vi "SNTP Light ActionVIs OnSave.vi"(8 "error in (no error)":errorcluster, 11 "Node Ptr":T1 format="%.0x") -> (0 "error out":errorcluster, 3 "Node Ptr 2":T1=18446744073709551615 format="%.0x")   [LabVIEW 2013, in "SNTP Light Custom Device Configuration.lvlib"]
uses:
  SNTP Light Custom Device Configuration.lvlib
  <vilib>/NI Veristand/Custom Device API/Custom Device API.lvlib
  NationalInstruments.VeriStand.SystemStorage
  NationalInstruments.VeriStand.SystemDefinitionAPI
  <vilib>/NI Veristand/Custom Device API/Custom Device Item Ref.ctl
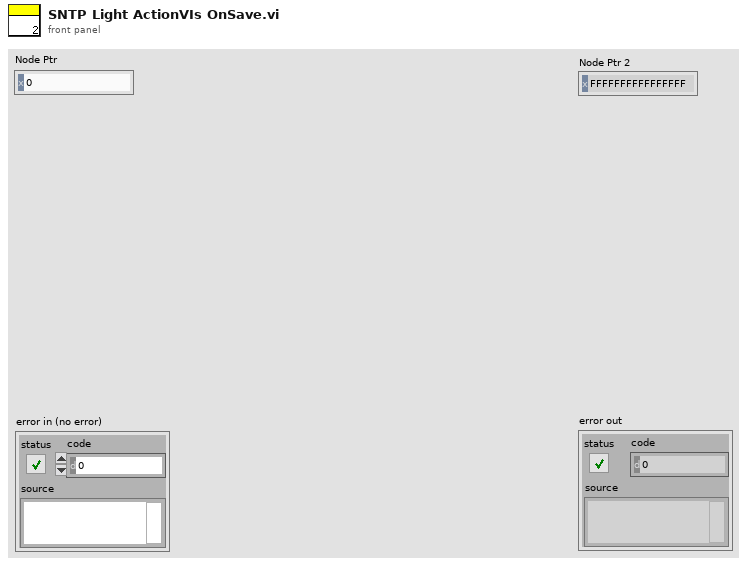
[diagram p1: front panel]
types:
  T1 = typedef "Custom Device API.lvlib/Custom Device Item Ref.ctl" = u64
  T2 = typedef "Custom Device API.lvlib/Custom Device Pointer.ctl" = refnum<k24>
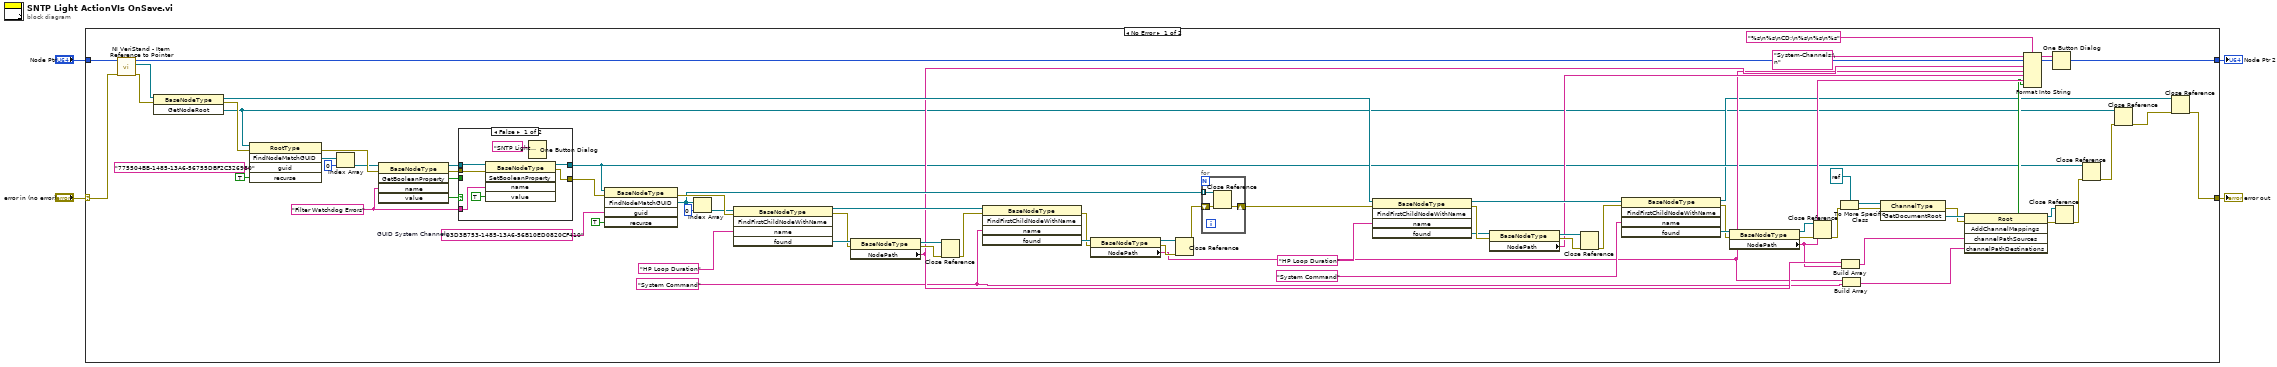
[diagram p0: block diagram]
diagram:
  n1 = case shown="No Error" "error in (no error)" {
    selector: "error in (no error)" -> [w79 w94]
    tunnel: [w74 w94] -> w3
    tunnel: "Node Ptr" -> [w80 w93]
    tunnel: [w76 w93] -> w1
    frame No Error {
      w16 = "System Command" ("name")
      w63 = "03D3B753-1485-13A6-56B10ED0820CF410"  # GUID System Channels
      w64 = "Filter Watchdog Errors" ("name")
      n2 = call <vilib>:"NI VeriStand - Item Reference to Pointer.vi"("error in (no error)"=w79, "Item Ref in"=w80) -> ("error out"=w77:errorcluster, "Node Pointer"=w78:T2, "Item Ref out"=w76:T1)  [unwired: 6 in, 1 out]
      n3 = invoke class="BaseNodeType" method="GetNodeRoot"(reference=w78, error in=w77) -> (reference out=w31:T2, error out=w73:errorcluster, "GetNodeRoot"=w5:refnum<k24>)  [unwired: 1 in]
      n4 = invoke class="RootType" method="FindNodeMatchGUID"(reference=w5, error in=w73, "guid"="775504BB-1485-13A6-56755DBF2C326980", "recurse"=TRUE) -> (error out=w70:errorcluster, "FindNodeMatchGUID"=w69:refnum<k24>[])  [unwired: 1 in, 3 out]
      n5 = Index Array(array=w69, index=0) -> (element=w28:refnum<k24>)
      n6 = invoke class="BaseNodeType" method="GetBooleanProperty"(reference=w28, error in=w70, "name"=w64) -> (reference out=w66:refnum<k24>, error out=w65:errorcluster, "GetBooleanProperty"=w75:bool, "value"=w67:bool)  [unwired: 2 in, 1 out]
      n7 = case shown="False" w67 {
        tunnel: w75 -> [_ _]
        tunnel: w66 -> [w90 w92]
        tunnel: [w89 w92] -> w13
        tunnel: w65 -> [w88 w91]
        tunnel: [w87 w91] -> w62
        tunnel: w64 -> [w86 _]
        frame False {
          n8 = invoke class="BaseNodeType" method="SetBooleanProperty"(reference=w90, error in=w88, "name"=w86, "value"=TRUE) -> (reference out=w89:refnum<k24>, error out=w87:errorcluster)  [unwired: 1 in, 3 out]
          n9 = One Button Dialog(message="SNTP Light Custom Device: \"Filter Watchdog Errors\" Controller Property forced to TRUE.") -> ()  [unwired: 1 in, 1 out]
        }
        frame True {
        }
      }
      n10 = invoke class="BaseNodeType" method="FindNodeMatchGUID"(reference=w13, error in=w62, "guid"=w63, "recurse"=TRUE) -> (error out=w59:errorcluster, "FindNodeMatchGUID"=w44:refnum<k24>[])  [unwired: 1 in, 3 out]
      n11 = Index Array(array=w44, index=0) -> (element=w30:refnum<k24>)
      n12 = invoke class="BaseNodeType" method="FindFirstChildNodeWithName"(reference=w30, error in=w59, "name"="HP Loop Duration") -> (reference out=w57:refnum<k24>, error out=w55:errorcluster, "found"=w56:refnum<k24>)  [unwired: 2 in, 2 out]
      n13 = property class="BaseNodeType"(reference=w56, error in=w55) -> (reference out=w54:refnum<k24>, error out=w53:errorcluster, "NodePath"=w18:string)
      n14 = Close Reference(reference=w54, error in (no error)=w53) -> (error out=w49:errorcluster)
      n15 = invoke class="BaseNodeType" method="FindFirstChildNodeWithName"(reference=w57, error in=w49, "name"=w16) -> (error out=w48:errorcluster, "found"=w50:refnum<k24>)  [unwired: 2 in, 3 out]
      n16 = property class="BaseNodeType"(reference=w50, error in=w48) -> (reference out=w51:refnum<k24>, error out=w52:errorcluster, "NodePath"=w17:string)
      n17 = Close Reference(reference=w51, error in (no error)=w52) -> (error out=w43:errorcluster)
      n18 = for {
        tunnel: w44 -> [w83] mode=indexing
        shift-right: [w81] -> w29
        shift-left: w43 -> [w82]
        n19 = Close Reference(reference=w83, error in (no error)=w82) -> (error out=w81:errorcluster)
      }
      n20 = invoke class="BaseNodeType" method="FindFirstChildNodeWithName"(reference=w31, error in=w29, "name"="HP Loop Duration") -> (reference out=w34:T2, error out=w37:errorcluster, "found"=w10:refnum<k24>)  [unwired: 2 in, 2 out]
      n21 = property class="BaseNodeType"(reference=w10, error in=w37) -> (reference out=w40:refnum<k24>, error out=w41:errorcluster, "NodePath"=w33:string)
      n22 = Close Reference(reference=w40, error in (no error)=w41) -> (error out=w36:errorcluster)
      n23 = invoke class="BaseNodeType" method="FindFirstChildNodeWithName"(reference=w34, error in=w36, "name"="System Command") -> (reference out=w12:T2, error out=w35:errorcluster, "found"=w42:refnum<k24>)  [unwired: 2 in, 2 out]
      n24 = property class="BaseNodeType"(reference=w42, error in=w35) -> (reference out=w6:refnum<k24>, error out=w8:errorcluster, "NodePath"=w15:string)
      n25 = Close Reference(reference=w6, error in (no error)=w8) -> (error out=w7:errorcluster)
      n26 = To More Specific Class(target class=refnum<k24> refnum, error in=w7) -> (specific class reference=w11:refnum<k24>, error out=w27:errorcluster)  [unwired: 1 in]
      n27 = Build Array(w18, w15) -> (w20:string[])
      n28 = Build Array(w17, w16) -> (w19:string[])
      n29 = invoke class="ChannelType" method="GetDocumentRoot"(reference=w11, error in=w27) -> (error out=w25:errorcluster, "GetDocumentRoot"=w26:refnum<k24>)  [unwired: 1 in, 1 out]
      n30 = invoke class="Root" method="AddChannelMappings"(reference=w26, error in=w25, "channelPathSources"=w20, "channelPathDestinations"=w19) -> (reference out=w23:refnum<k24>, error out=w24:errorcluster, "AddChannelMappings"=w14:bool)  [unwired: 1 in, 2 out]
      n31 = Format Into String(format string="%s\n%s\nCD:\n%s\n%s\n%s", initial string="System-Channels:\n", w18, w17, w33, w15, w14) -> (resulting string=w47:string)  [unwired: 1 in, 1 out]
      n32 = One Button Dialog(message=w47) -> ()  [unwired: 1 in, 1 out]
      n33 = Close Reference(reference=w23, error in (no error)=w24) -> (error out=w22:errorcluster)
      n34 = Close Reference(reference=w13, error in (no error)=w22) -> (error out=w21:errorcluster)
      n35 = Close Reference(reference=w5, error in (no error)=w21) -> (error out=w32:errorcluster)
      n36 = Close Reference(reference=w12, error in (no error)=w32) -> (error out=w74:errorcluster)
    }
    frame Error {
    }
  }
  "error out" <- w3
  "Node Ptr 2" <- w1
